vi "format data.vi"(8 "error in (no error)":errorcluster, 10 "Data Array":dbl[][](array[numeric]), 11 "Date/Time Array":timestamp[](array[timestamp])) -> (0 "error out":errorcluster, 2 "Data":string[][](array[string]))   [LabVIEW 2025, in "Data Log.lvclass"]
uses:
  Data Log.lvclass
  Data Log.lvclass/Data Log.ctl
panel:
  in  "Data 2":string[][](array[string])
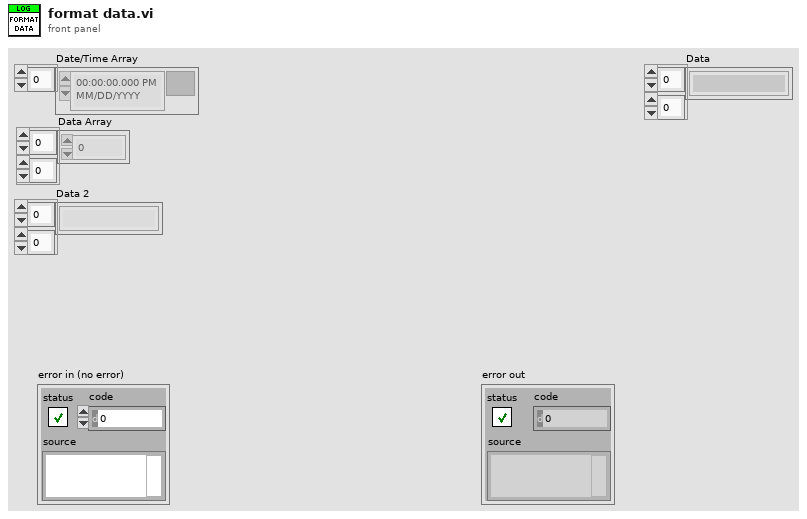
[diagram p1: front panel]
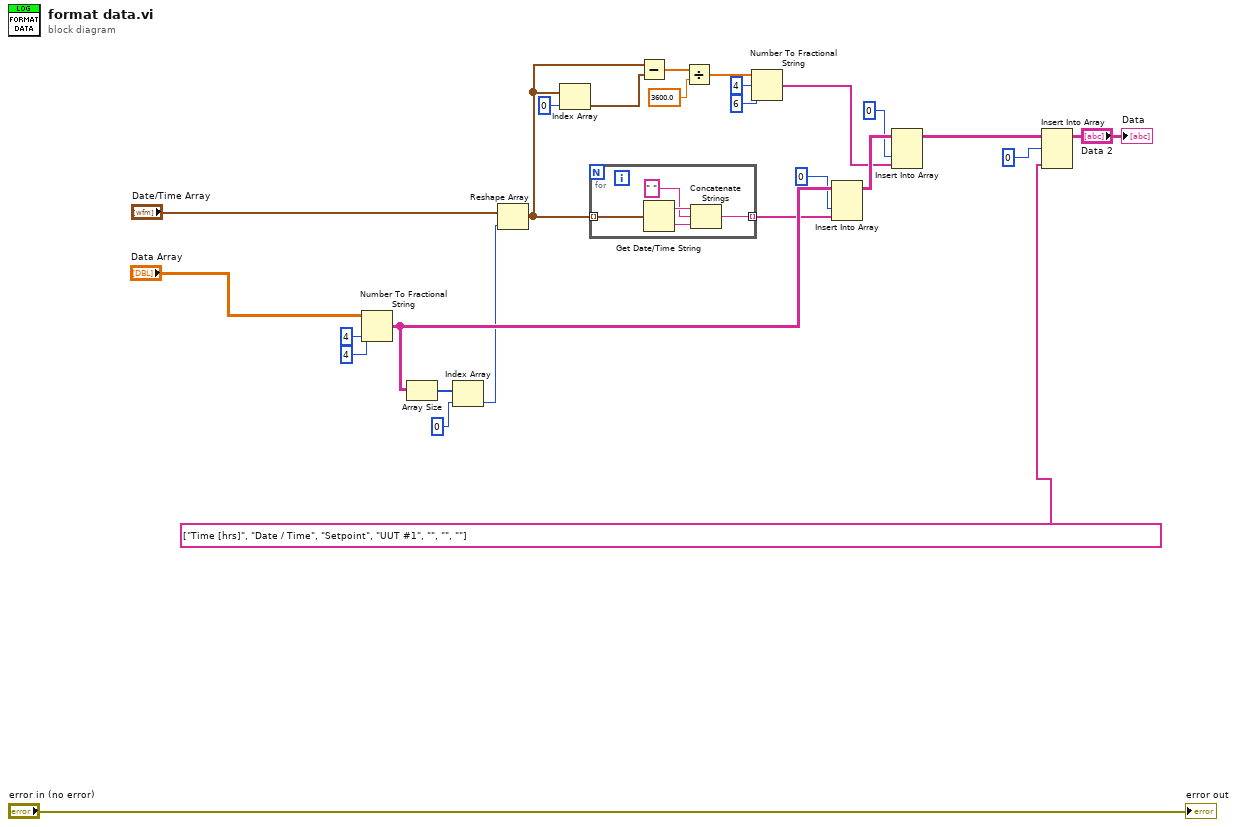
[diagram p0: block diagram]
diagram:
  n1 = Number To Fractional String(number="Data Array", width (-)=i16 4, precision (6)=i16 4) -> (F-format string=w25:string[][])  [unwired: 1 in]
  n2 = Array Size(array=w25) -> (size(s)=w20:i32[])
  n3 = Index Array(array=w20, index=0) -> (element=w22:i32)
  n4 = Reshape Array("Date/Time Array", w22) -> (w16:timestamp[])
  n5 = Index Array(array=w16, index=0) -> (element=w15:timestamp)
  n6 = for {
    tunnel: w16 -> [w31] mode=indexing
    tunnel: [w29] -> w23 mode=indexing
    n7 = Get Date/Time String(seconds (now)=w31) -> (date string=w28:string, time string=w30:string)  [unwired: 2 in]
    n8 = Concatenate Strings(w28, " ", w30) -> (w29:string)
  }
  n9 = Subtract(x=w16, y=w15) -> (x-y=w14:dbl[])
  n10 = Divide(x=w14, y=3600.0) -> (x/y=w12:dbl[])
  n11 = Number To Fractional String(number=w12, width (-)=i16 4, precision (6)=i16 6) -> (F-format string=w8:string[])  [unwired: 1 in]
  n12 = Insert Into Array(array=w25, index (col)=0 ("index (row)"), new element=w23) -> (w9:string[][])  [unwired: 1 in]
  n13 = Insert Into Array(array=w9, index (col)=0 ("disabled index (col)"), new element=w8) -> (w6:string[][])  [unwired: 1 in]
  n14 = Insert Into Array(array=w6, index (row)=0, new element=string[] ["Time [hrs]", "Date / Time", "Setpoint", "UUT #1", "", "", ""]) -> (→"Data":string[][])  [unwired: 1 in]
  "error out" <- "error in (no error)"
